vi "HDF5_Write_Validity_record.vi"(4 "RedundantFile":i32, 5 "WeatherStatus":bool[](array[boolean]), 6 "Alarm Status":T1, 7 "SaturationStatus":T2, 8 "error in":errorcluster, 9 "AllAlarms":T3[](array[typedef]), 10 "LogData":T4 {"NoiseInfo"."HDF5_NoiseInfo"."Sum" format="%^#.1g"}, 11 "ValidRef":T19 {"Alarm_Source_dset" format="%.0x"; "Time_AlarmChange_dset" format="%.0x"; "Time_Valid_dset" format="%.0x"; "Alarm_Valid_dset" format="%.0x"; "Saturat_dset" format="%.0x"; "Group_ref" format="%.0x"; "Weath_Valid_dset" format="%.0x"; "Disdr_Valid_dset" format="%.0x"}) -> (0 "error out":errorcluster)   [LabVIEW 2018]
doc: "Write a single Tone<x> record with timestamp:\nTone1\n Beac - cluster\n BeacZoom - 1024 element Double array (waveform) \n Cal - cluster\n CalZoom - 1024 element Double array (waveform)"
uses:
  HDF5_Validty_refs.ctl
  <vilib>/addons/h5labview2/base/hid_t.ctl
  Controls/Clusts/LogDataClust.ctl
  Controls/Clusts/ToneLogBuffered.ctl
  Controls/Enums/TargetNumber.ctl
  Controls/Clusts/SaturationMonitorBuffer.ctl
  TC_Data_Structure.ctl
  Controls/Clusts/AI_Clust.ctl
  HDF5_NoiseInfoClust.ctl
  DisdrometerData.ctl
  DisdromterSummaryData.ctl
  Disdrometer/Disdrometer_Status_Cluster.ctl
  Controls/Clusts/WeatherDataClust.ctl
  Controls/Clusts/ValidityWeatherClust.ctl
  Controls/Clusts/TE_Data_Clust.ctl
  HDF5_ADAM_Data.ctl
  Controls/Clusts/TimeDomainData.ctl
  Controls/Clusts/ErrorStatus.ctl
  Controls/Clusts/Saturation_Status_Clust.ctl
  Controls/Clusts/DigOutClust.ctl
  <vilib>/addons/h5labview2/base/lib_path.vi
  <vilib>/addons/h5labview2/base/H5Equery.vi
  <vilib>/addons/h5labview2/dataset/H5Dwrite.llb/H5Dwrite.xnode
  <vilib>/addons/h5labview2/dataset/H5D.lvlib
  <vilib>/addons/h5labview2/space/H5S.lvlib
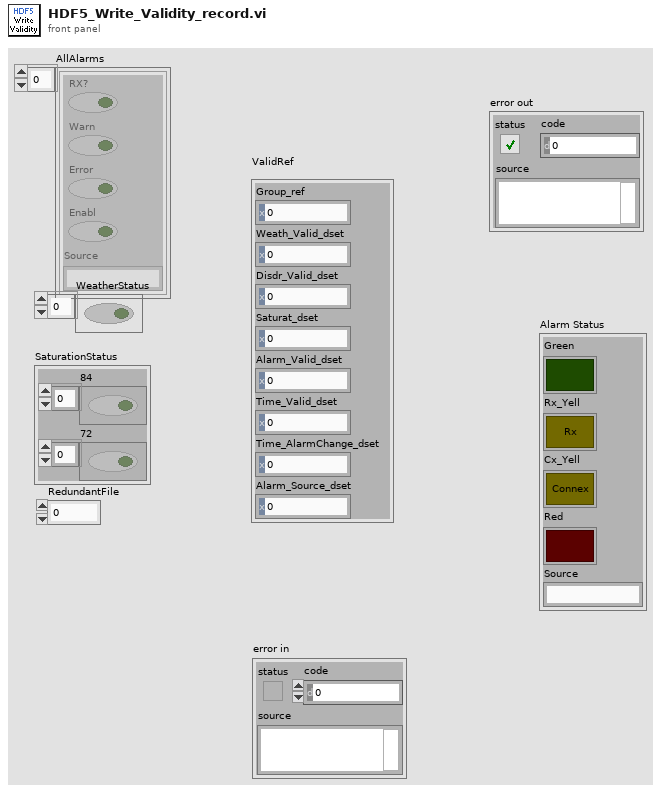
[diagram p1: front panel]
types:
  T1 = typedef "DigOutClust.ctl" = cluster{"Green":bool, "Rx_Yell":bool, "Cx_Yell":bool, "Red":bool, "Source":string}
  T2 = typedef "Saturation_Status_Clust.ctl" = cluster{"84":bool[], "72":bool[]}
  T3 = typedef "ErrorStatus.ctl" = cluster{"RX?":bool, "Warn":bool, "Error":bool, "Enabl":bool, "Source":string}
  T4 = typedef "LogDataClust.ctl" = cluster{"Tone":T5[], "TCData":T8, "AI":T9, "NoiseTrace":cluster{"Target":T6, "NoiseTrace":dbl[]}[], "NoiseInfo":cluster{"Target":T6, "HDF5_NoiseInfo":T10}[], "Disdrom":T11[], "Weath":T14[], "TE":T16, "ADAM":T17, "TimeDomain":T18[]}
  T5 = typedef "ToneLogBuffered.ctl" = cluster{"Count":i32, "CalVal":sgl[], "CalLoc":i32[], "BeacVal":sgl[], "BeacLoc":i32[], "BeacShift":i32[], "Enum":T6, "df":dbl, "PwrSpectr":sgl[][], "ISpectr":sgl[][], "QSpectr":sgl[][], "Time":timestamp[], "SNR":sgl[], "AboveThresh":bool[], "10Hz_PeakVal":dbl[], "Phase":sgl[], "DeltaPhase":dbl[], "Saturat":T7, "10MHz":bool}
  T6 = typedef "TargetNumber.ctl" = enum16{"1", "2", "3", "4"}
  T7 = typedef "SaturationMonitorBuffer.ctl" = cluster{"Meas":bool[], "Stage1":bool[], "Stage4":bool[], "Stage5":bool[], "Stage6":bool[], "Stage7":bool[]}
  T8 = typedef "TC_Data_Structure.ctl" = cluster{"TimeStamp":dbl, "TimeString":string, "TC0_LP1_Hi":dbl, "TC1_LP1_MidHi":dbl, "TC2_LP1_Mid":dbl, "TC3_LP1_LoMid":dbl, "TC4_LP1_Lo":dbl, "TC5_LP2_Hi":dbl, "TC6_LP2_MidHi":dbl, "TC7_LP2_Mid":dbl, "TC8_LP2_LoMid":dbl, "TC9_LP2_Lo":dbl, "TC10_HVAC_Cond_In":dbl, "TC11_HVAC_Cond_Out":dbl, "TC12_Gen_Exhaust":dbl, "TC13_Amb_Inter":dbl, "TC14_Unused":dbl, "TC15_Unused":dbl, "TC16_Unused":dbl, "TC17_Unused":dbl, "TC18_Unused":dbl, "TC19_Unused":dbl, "TC20_Unused":dbl, "TC21_Unused":dbl, "TC22_Unused":dbl, "TC23_Unused":dbl, "TC24_Unused":dbl, "TC25_Unused":dbl, "TC26_Unused":dbl, "TC27_Unused":dbl, "TC28_Unused":dbl, "TC29_Unused":dbl, "TC30_Unused":dbl, "TC31_Unused":dbl}
  T9 = typedef "AI_Clust.ctl" = cluster{"TimeString":string, "Time Stamp":dbl, "AI0_Unused":dbl, "AI1_-5V":dbl, "AI2_+5V":dbl, "AI3_+6V":dbl, "AI4_+12V":dbl, "AI5_+15V":dbl, "AI6_+28V":dbl, "AI7_Unused":dbl, "Ai16_72GHz_CalPower":dbl, "Ai17_84GHz_CalPower":dbl, "Ai18_InclinAz":dbl, "Ai19_InclinEl":dbl, "Ai20_BlowerPwr":dbl, "Ai21_Unused":dbl, "Ai22_Unused":dbl, "Ai23_Unused":dbl, "InclinA_StdDev":dbl, "InclinB_StdDev":dbl, "InclinAz_Unfilt":dbl, "InclinEl_Unfilt":dbl}
  T10 = typedef "HDF5_NoiseInfoClust.ctl" = cluster{"Timestring":string, "Timestamp":dbl, "df":dbl, "Sum":dbl}
  T11 = typedef "DisdrometerData.ctl" = cluster{"Spectrum Data":i16[], "DisdromSummary":T12, "Status":T13}
  T12 = typedef "DisdromterSummaryData.ctl" = cluster{"current time":dbl, "Timestamp":dbl, "Total Rain Rate":dbl, "Liquid Rain Rate":dbl, "Solid Rain Rate":dbl, "Total Rainfall":dbl, "Visibility":dbl, "Radar Reflectivity":dbl, "Max Diameter Hail":dbl, "Measured Particles":i32, "Particle Min Speed":i16, "Particle Max Speed":i16, "Particle Min Diam":i16, "NonHydr Particles":i16, "NonHydr Volume":dbl, "Unkn Particles":i16, "Unkn Volume":dbl, "HydroType":i8}
  T13 = typedef "Disdrometer_Status_Cluster.ctl" = cluster{"Laser":bool, "Signal":bool, "LaserTemp_Analog":bool, "LaserTemp_Digital":bool, "LaserCurrent_Analog":bool, "LaserCurrent_Digital":bool, "SensorSupply":bool, "HeatLaserHead":bool, "HeatReceiverHead":bool, "TempSensor":bool, "HeatSupply":bool, "HeatHousing":bool, "HeatHeads":bool, "HeatCarriers":bool, "OutputLaserPower":bool, "Checksum":bool, "StatusInt":u16}
  T14 = typedef "WeatherDataClust.ctl" = cluster{"TimeString":string, "Timestamp":dbl, "Wind Speed":sgl, "Wind Gusts":sgl, "Wind Dir":sgl, "Wind Dir STD":sgl, "Temperature":sgl, "Humidity":sgl, "Pressure":sgl, "Rain Rate":i16, "Rain Fall":sgl, "Status":T15}
  T15 = typedef "ValidityWeatherClust.ctl" = cluster{"Temp_OutOfBounds":bool, "Temp_IncrSTD":bool, "Temp_Oth":bool, "BarPress_OutOfBounds":bool, "BarPress_IncrSTD":bool, "BarPress_Change":bool, "BarPress_Other":bool, "Humid_OutOfBounds":bool, "Humid_IncrSTD":bool, "Humid_Other":bool, "Wind__Spd_OutOfBounds":bool, "Wind_Dir_OutOfBounds":bool, "RainBuck_OutOfBounds":bool, "RainBuck_Disdrom":bool, "Disdrom_RainBuck":bool, "Placeholder":bool}
  T16 = typedef "TE_Data_Clust.ctl" = cluster{"TimeString":string, "TimeStamp":dbl, "Temp":dbl, "Output":dbl, "Temp 2":dbl, "Output 2":dbl, "Temp 3":dbl, "Output 3":dbl}
  T17 = typedef "HDF5_ADAM_Data.ctl" = cluster{"Timestamp":dbl, "Time string":string, "Fault 1":bool, "Fault 2":bool, "Fault 3":bool, "Fault 4":bool, "Fault 5":bool, "Fault 6":bool, "Value 1":dbl, "Value 2":dbl, "Value 3":dbl, "Value 4":dbl, "Value 5":dbl, "Value 6":dbl}
  T18 = typedef "TimeDomainData.ctl" = cluster{"CalTimeVal":dbl[], "CalTimeCount":u32[], "Enum":T6}
  T19 = typedef "HDF5_Validty_refs.ctl" = cluster{"Group_ref":T20, "Weath_Valid_dset":T20, "Disdr_Valid_dset":T20, "Saturat_dset":T20, "Alarm_Valid_dset":T20, "Time_Valid_dset":T20, "Time_AlarmChange_dset":T20, "Alarm_Source_dset":T20}
  T20 = typedef "hid_t.ctl" = i32
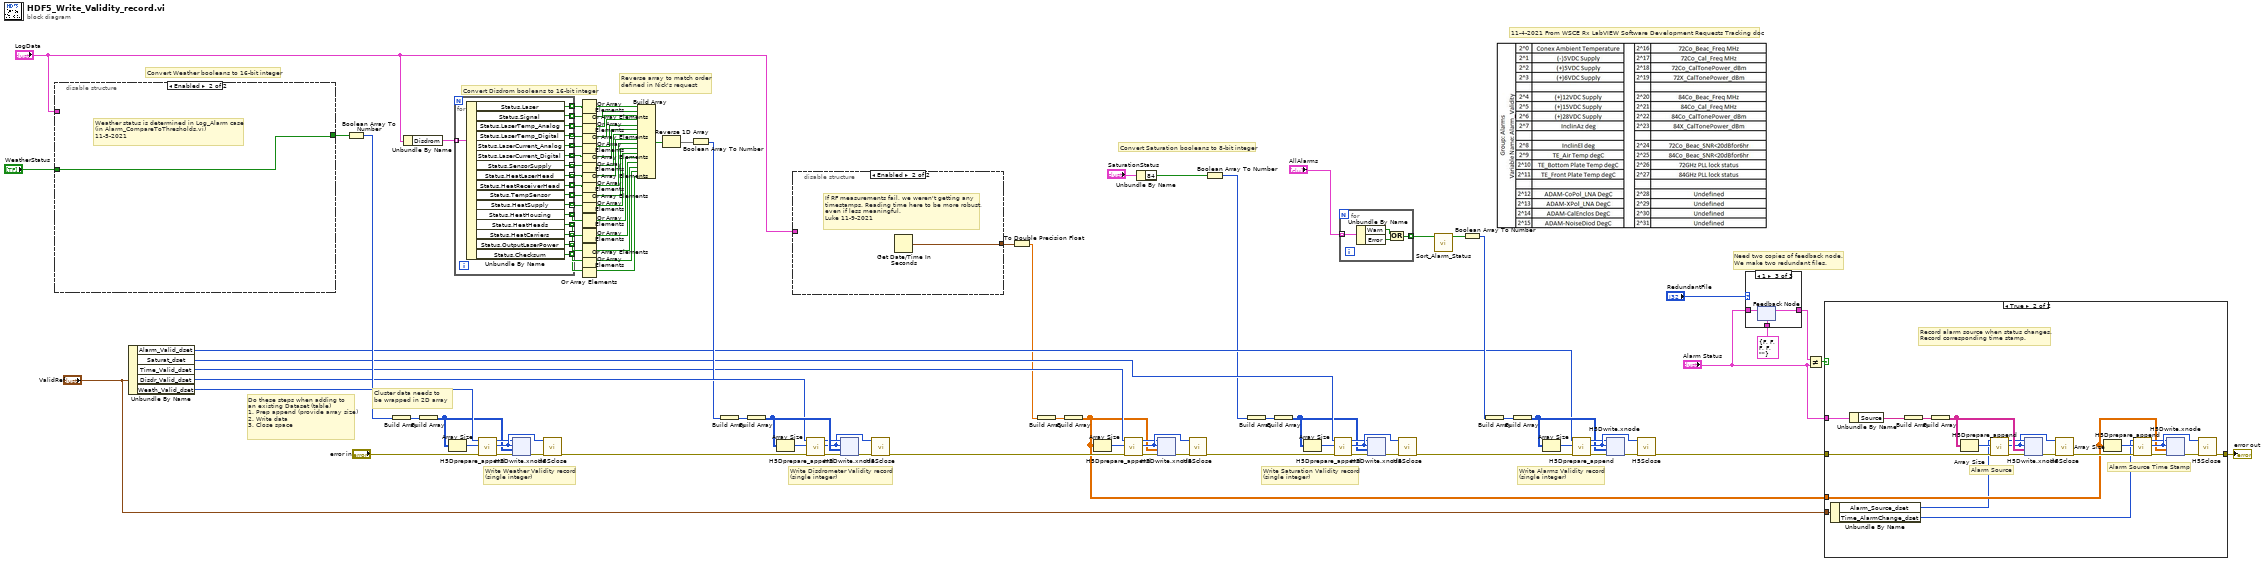
[diagram p0: block diagram]
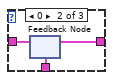
[diagram p3: hidden frame]
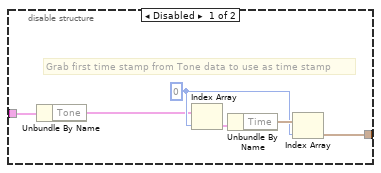
[diagram p4: hidden frame]
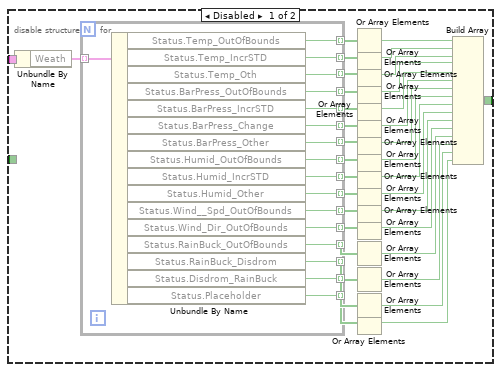
[diagram p6: hidden frame]
diagram:
  # "Need two copies of feedback node.\nWe make two redundant files."
  # "11-4-2021 From WSCE Rx LabVIEW Software Development Requests Tracking doc"
  # "Reverse array to match order defined in Nick's request"
  # "Write Alarms Validity record\n(single integer)"
  # "Write Saturation Validity record\n(single integer)"
  # "Write Disdrometer Validity record\n(single integer)"
  # "Convert Saturation booleans to 8-bit integer"
  # "Convert Disdrom booleans to 16-bit integer"
  # "Convert Weather booleans to 16-bit integer"
  # "Cluster data needs to \nbe wrapped in 2D array"
  # "Do these steps when adding to \nan existing Dataset (table)\n1. Prep append (provide array size)\n2. Write data\n3. Close space"
  # "Write Weather Validity record\n(single integer)"
  n1 = disable-structure shown="Enabled" {
    disable-tunnel: [w104 w155] -> w93
    disable-tunnel: "LogData" -> [w103 _]
    disable-tunnel: "WeatherStatus" -> [_ w155]
    frame Disabled {
      n2 = Unbundle By Name(w103) -> ("Weath"=w137:T14[])
      n3 = for {
        tunnel: w137 -> [w154] mode=indexing
        tunnel: [w153] -> w136 mode=indexing
        tunnel: [w152] -> w135 mode=indexing
        tunnel: [w151] -> w134 mode=indexing
        tunnel: [w150] -> w133 mode=indexing
        tunnel: [w149] -> w132 mode=indexing
        tunnel: [w148] -> w131 mode=indexing
        tunnel: [w147] -> w130 mode=indexing
        tunnel: [w146] -> w129 mode=indexing
        tunnel: [w145] -> w128 mode=indexing
        tunnel: [w144] -> w127 mode=indexing
        tunnel: [w143] -> w126 mode=indexing
        tunnel: [w142] -> w125 mode=indexing
        tunnel: [w141] -> w124 mode=indexing
        tunnel: [w140] -> w123 mode=indexing
        tunnel: [w139] -> w122 mode=indexing
        tunnel: [w138] -> w121 mode=indexing
        n4 = Unbundle By Name(w154) -> ("Status.Temp_OutOfBounds"=w153:bool, "Status.Temp_IncrSTD"=w152:bool, "Status.Temp_Oth"=w151:bool, "Status.BarPress_OutOfBounds"=w150:bool, "Status.BarPress_IncrSTD"=w149:bool, "Status.BarPress_Change"=w148:bool, "Status.BarPress_Other"=w147:bool, "Status.Humid_OutOfBounds"=w146:bool, "Status.Humid_IncrSTD"=w145:bool, "Status.Humid_Other"=w144:bool, "Status.Wind__Spd_OutOfBounds"=w143:bool, "Status.Wind_Dir_OutOfBounds"=w142:bool, "Status.RainBuck_OutOfBounds"=w141:bool, "Status.RainBuck_Disdrom"=w140:bool, "Status.Disdrom_RainBuck"=w139:bool, "Status.Placeholder"=w138:bool)
      }
      n5 = Or Array Elements(Boolean array=w136) -> (logical OR=w120:bool)
      n6 = Or Array Elements(Boolean array=w135) -> (logical OR=w119:bool)
      n7 = Or Array Elements(Boolean array=w134) -> (logical OR=w118:bool)
      n8 = Or Array Elements(Boolean array=w133) -> (logical OR=w117:bool)
      n9 = Or Array Elements(Boolean array=w132) -> (logical OR=w116:bool)
      n10 = Or Array Elements(Boolean array=w131) -> (logical OR=w115:bool)
      n11 = Or Array Elements(Boolean array=w130) -> (logical OR=w114:bool)
      n12 = Or Array Elements(Boolean array=w129) -> (logical OR=w113:bool)
      n13 = Or Array Elements(Boolean array=w128) -> (logical OR=w112:bool)
      n14 = Or Array Elements(Boolean array=w127) -> (logical OR=w111:bool)
      n15 = Or Array Elements(Boolean array=w126) -> (logical OR=w110:bool)
      n16 = Or Array Elements(Boolean array=w125) -> (logical OR=w109:bool)
      n17 = Or Array Elements(Boolean array=w124) -> (logical OR=w108:bool)
      n18 = Or Array Elements(Boolean array=w123) -> (logical OR=w107:bool)
      n19 = Or Array Elements(Boolean array=w122) -> (logical OR=w106:bool)
      n20 = Or Array Elements(Boolean array=w121) -> (logical OR=w105:bool)
      n21 = Build Array(w120, w119, w118, w117, w116, w115, w114, w113, w112, w111, w110, w109, w108, w107, w106, w105) -> (w104:bool[])
    }
    frame Enabled {
      # "Weather status is determined in Log_Alarm case \n(in Alarm_CompareToThresholds.vi)\n11-5-2021"
    }
  }
  n22 = Unbundle By Name("ValidRef") -> ("Alarm_Valid_dset"=w37:T20, "Saturat_dset"=w38:T20, "Time_Valid_dset"=w17:T20, "Disdr_Valid_dset"=w50:T20, "Weath_Valid_dset"=w98:T20)
  n23 = Boolean Array To Number(Boolean array=w93) -> (number=w92:u16)
  n24 = Build Array(w92) -> (w97:u16[])
  n25 = Unbundle By Name("LogData") -> ("Disdrom"=w83:T11[])
  n26 = Build Array(w97) -> (w96:u16[][])
  n27 = Array Size(array=w96) -> (size(s)=w95:i32[])
  n28 = for {
    tunnel: w83 -> [w172] mode=indexing
    tunnel: [w171] -> w66 mode=indexing
    tunnel: [w170] -> w65 mode=indexing
    tunnel: [w169] -> w64 mode=indexing
    tunnel: [w168] -> w63 mode=indexing
    tunnel: [w167] -> w62 mode=indexing
    tunnel: [w166] -> w61 mode=indexing
    tunnel: [w165] -> w60 mode=indexing
    tunnel: [w164] -> w59 mode=indexing
    tunnel: [w163] -> w58 mode=indexing
    tunnel: [w162] -> w57 mode=indexing
    tunnel: [w161] -> w56 mode=indexing
    tunnel: [w160] -> w55 mode=indexing
    tunnel: [w159] -> w54 mode=indexing
    tunnel: [w158] -> w53 mode=indexing
    tunnel: [w157] -> w52 mode=indexing
    tunnel: [w156] -> w51 mode=indexing
    n29 = Unbundle By Name(w172) -> ("Status.Laser"=w171:bool, "Status.Signal"=w170:bool, "Status.LaserTemp_Analog"=w169:bool, "Status.LaserTemp_Digital"=w168:bool, "Status.LaserCurrent_Analog"=w167:bool, "Status.LaserCurrent_Digital"=w166:bool, "Status.SensorSupply"=w165:bool, "Status.HeatLaserHead"=w164:bool, "Status.HeatReceiverHead"=w163:bool, "Status.TempSensor"=w162:bool, "Status.HeatSupply"=w161:bool, "Status.HeatHousing"=w160:bool, "Status.HeatHeads"=w159:bool, "Status.HeatCarriers"=w158:bool, "Status.OutputLaserPower"=w157:bool, "Status.Checksum"=w156:bool)
  }
  n30 = call <vilib>:"H5Dprepare_append.vi"("error in (no error)"="error in", "append dims"=w95, "dset in"=w98) -> ("error out"=w102:errorcluster, "space out"=w101:T20, "dset out"=w100:T20)  [unwired: 5 in, 1 out]
  n31 = xnode "H5Dwrite.xnode"("error in (no error)"=w102, "data"=w96, "file space"=w101, "ref in"=w100) -> ("error out"=w94:errorcluster)  [unwired: 3 in, 2 out]
  n32 = call <vilib>:"H5Sclose.vi"("error in (no error)"=w94, "space in"=w101) -> ("error out"=w86:errorcluster)  [unwired: 9 in]
  n33 = Or Array Elements(Boolean array=w66) -> (logical OR=w67:bool)
  n34 = Or Array Elements(Boolean array=w65) -> (logical OR=w68:bool)
  n35 = Or Array Elements(Boolean array=w64) -> (logical OR=w69:bool)
  n36 = Or Array Elements(Boolean array=w63) -> (logical OR=w70:bool)
  n37 = Or Array Elements(Boolean array=w62) -> (logical OR=w71:bool)
  n38 = Or Array Elements(Boolean array=w61) -> (logical OR=w72:bool)
  n39 = Or Array Elements(Boolean array=w60) -> (logical OR=w73:bool)
  n40 = Or Array Elements(Boolean array=w59) -> (logical OR=w74:bool)
  n41 = Or Array Elements(Boolean array=w58) -> (logical OR=w75:bool)
  n42 = Or Array Elements(Boolean array=w57) -> (logical OR=w76:bool)
  n43 = Or Array Elements(Boolean array=w56) -> (logical OR=w77:bool)
  n44 = Or Array Elements(Boolean array=w55) -> (logical OR=w78:bool)
  n45 = Or Array Elements(Boolean array=w54) -> (logical OR=w79:bool)
  n46 = Or Array Elements(Boolean array=w53) -> (logical OR=w80:bool)
  n47 = Or Array Elements(Boolean array=w52) -> (logical OR=w81:bool)
  n48 = Or Array Elements(Boolean array=w51) -> (logical OR=w82:bool)
  n49 = Build Array(w67, w68, w69, w70, w71, w72, w73, w74, w75, w76, w77, w78, w79, w80, w81, w82) -> (w49:bool[])
  n50 = Reverse 1D Array(array=w49) -> (reversed array=w28:bool[])
  n51 = Boolean Array To Number(Boolean array=w28) -> (number=w48:u16)
  n52 = Build Array(w48) -> (w89:u16[])
  n53 = Build Array(w89) -> (w90:u16[][])
  n54 = Array Size(array=w90) -> (size(s)=w91:i32[])
  n55 = disable-structure shown="Enabled" {
    disable-tunnel: "LogData" -> [w175 _]
    disable-tunnel: [w173 w179] -> w18
    frame Disabled {
      w176 = 0 ("index")
      # "Grab first time stamp from Tone data to use as time stamp"
      n56 = Unbundle By Name(w175) -> ("Tone"=w174:T5[])
      n57 = Index Array(array=w174, index=w176) -> (element=w178:T5)
      n58 = Unbundle By Name(w178) -> ("Time"=w177:timestamp[])
      n59 = Index Array(array=w177, index=w176) -> (element=w173:timestamp)
    }
    frame Enabled {
      # "If RF measurements fail, we weren't getting any\ntimestamps. Reading time here to be more robust,\neven if less meaningful.\nLuke 11-9-2021"
      n60 = Get Date/Time In Seconds() -> (seconds since 1Jan1904=w179:timestamp)
    }
  }
  n61 = call <vilib>:"H5Dprepare_append.vi"("error in (no error)"=w86, "append dims"=w91, "dset in"=w50) -> ("error out"=w85:errorcluster, "space out"=w87:T20, "dset out"=w88:T20)  [unwired: 5 in, 1 out]
  n62 = xnode "H5Dwrite.xnode"("error in (no error)"=w85, "data"=w90, "file space"=w87, "ref in"=w88) -> ("error out"=w84:errorcluster)  [unwired: 3 in, 2 out]
  n63 = call <vilib>:"H5Sclose.vi"("error in (no error)"=w84, "space in"=w87) -> ("error out"=w22:errorcluster)  [unwired: 9 in]
  n64 = To Double Precision Float(number=w18) -> (double precision float=w16:dbl)
  n65 = Build Array(w16) -> (w24:dbl[])
  n66 = Build Array(w24) -> (w2:dbl[][])
  n67 = Array Size(array=w2) -> (size(s)=w23:i32[])
  n68 = call <vilib>:"H5Dprepare_append.vi"("error in (no error)"=w22, "append dims"=w23, "dset in"=w17) -> ("error out"=w21:errorcluster, "space out"=w26:T20, "dset out"=w25:T20)  [unwired: 5 in, 1 out]
  n69 = Unbundle By Name("SaturationStatus") -> ("84"=w14:bool[])
  n70 = xnode "H5Dwrite.xnode"("error in (no error)"=w21, "data"=w2, "file space"=w26, "ref in"=w25) -> ("error out"=w20:errorcluster)  [unwired: 3 in, 2 out]
  n71 = call <vilib>:"H5Sclose.vi"("error in (no error)"=w20, "space in"=w26) -> ("error out"=w19:errorcluster)  [unwired: 9 in]
  n72 = Boolean Array To Number(Boolean array=w14) -> (number=w29:u8)
  n73 = Build Array(w29) -> (w34:u8[])
  n74 = Build Array(w34) -> (w4:u8[][])
  n75 = Array Size(array=w4) -> (size(s)=w33:i32[])
  n76 = call <vilib>:"H5Dprepare_append.vi"("error in (no error)"=w19, "append dims"=w33, "dset in"=w38) -> ("error out"=w32:errorcluster, "space out"=w36:T20, "dset out"=w35:T20)  [unwired: 5 in, 1 out]
  n77 = for {
    tunnel: "AllAlarms" -> [w181] mode=indexing
    tunnel: [w180] -> w13 mode=indexing
    n78 = Unbundle By Name(w181) -> ("Warn"=w183:bool, "Error"=w182:bool)
    n79 = Or(x=w183, y=w182) -> (x .or. y?=w180:bool)
  }
  n80 = xnode "H5Dwrite.xnode"("error in (no error)"=w32, "data"=w4, "file space"=w36, "ref in"=w35) -> ("error out"=w31:errorcluster)  [unwired: 3 in, 2 out]
  n81 = call <vilib>:"H5Sclose.vi"("error in (no error)"=w31, "space in"=w36) -> ("error out"=w30:errorcluster)  [unwired: 9 in]
  n82 = call "Sort_Alarm_Status.vi"("Array in"=w13) -> ("Array out"=w12:bool[])  [unwired: 10 in]
  n83 = Boolean Array To Number(Boolean array=w12) -> (number=w39:u32)
  n84 = Build Array(w39) -> (w42:u32[])
  n85 = Build Array(w42) -> (w41:u32[][])
  n86 = Array Size(array=w41) -> (size(s)=w40:i32[])
  n87 = call <vilib>:"H5Dprepare_append.vi"("error in (no error)"=w30, "append dims"=w40, "dset in"=w37) -> ("error out"=w45:errorcluster, "space out"=w44:T20, "dset out"=w43:T20)  [unwired: 5 in, 1 out]
  n88 = xnode "H5Dwrite.xnode"("error in (no error)"=w45, "data"=w41, "file space"=w44, "ref in"=w43) -> ("error out"=w46:errorcluster)  [unwired: 3 in, 2 out]
  n89 = call <vilib>:"H5Sclose.vi"("error in (no error)"=w46, "space in"=w44) -> ("error out"=w10:errorcluster)  [unwired: 9 in]
  n90 = case shown="1" "RedundantFile" {
    tunnel: T1 {"Green"=FALSE, "Rx_Yell"=FALSE, "Cx_Yell"=FALSE, "Red"=FALSE, "Source"=""} ("Alarm Status") -> [_ w187 w190]
    tunnel: [w184 w186 w189] -> w7
    tunnel: "Alarm Status" -> [w184 w185 w188]
    frame Default {
    }
    frame 0 {
      n91 = feedback #1(w187) -> (w186:T1)
      n92 = feedback-in #1(w185) -> ()
    }
    frame 1 {
      n93 = feedback #2(w190) -> (w189:T1)
      n94 = feedback-in #2(w188) -> ()
    }
  }
  n95 = Not Equal?(x=w7, y="Alarm Status") -> (x != y?=w6:bool)
  n96 = case shown="True" w6 {
    tunnel: w10 -> [w191 w205]
    tunnel: [w191 w198] -> w9
    tunnel: "Alarm Status" -> [_ w192]
    tunnel: w2 -> [_ w197]
    tunnel: "ValidRef" -> [_ w196]
    frame False {
    }
    frame True {
      # "Record alarm source when status changes.\nRecord corresponding time stamp."
      # "Alarm Source Time Stamp"
      # "Alarm Source"
      n97 = Unbundle By Name(w196) -> ("Alarm_Source_dset"=w195:T20, "Time_AlarmChange_dset"=w194:T20)
      n98 = Unbundle By Name(w192) -> ("Source"=w193:string)
      n99 = Build Array(w193) -> (w210:string[])
      n100 = Build Array(w210) -> (w211:string[][])
      n101 = Array Size(array=w211) -> (size(s)=w212:i32[])
      n102 = call <vilib>:"H5Dprepare_append.vi"("error in (no error)"=w205, "append dims"=w212, "dset in"=w195) -> ("error out"=w207:errorcluster, "space out"=w208:T20, "dset out"=w209:T20)  [unwired: 5 in, 1 out]
      n103 = xnode "H5Dwrite.xnode"("error in (no error)"=w207, "data"=w211, "file space"=w208, "ref in"=w209) -> ("error out"=w206:errorcluster)  [unwired: 3 in, 2 out]
      n104 = call <vilib>:"H5Sclose.vi"("error in (no error)"=w206, "space in"=w208) -> ("error out"=w199:errorcluster)  [unwired: 9 in]
      n105 = Array Size(array=w197) -> (size(s)=w200:i32[])
      n106 = call <vilib>:"H5Dprepare_append.vi"("error in (no error)"=w199, "append dims"=w200, "dset in"=w194) -> ("error out"=w203:errorcluster, "space out"=w202:T20, "dset out"=w201:T20)  [unwired: 5 in, 1 out]
      n107 = xnode "H5Dwrite.xnode"("error in (no error)"=w203, "data"=w197, "file space"=w202, "ref in"=w201) -> ("error out"=w204:errorcluster)  [unwired: 3 in, 2 out]
      n108 = call <vilib>:"H5Sclose.vi"("error in (no error)"=w204, "space in"=w202) -> ("error out"=w198:errorcluster)  [unwired: 9 in]
    }
  }
  "error out" <- w9
